vi "Configure Status.vi"(0 "disk streaming in":refnum<class "Disk Streaming.lvclass">, 1 "preview size (samples)":u32, 5 "error in (no error)":errorcluster) -> (14 "disk streaming out":refnum<class "Disk Streaming.lvclass">, 19 "error out":errorcluster)   [LabVIEW 2021, in "Disk Streaming.lvclass"]
doc: "Configures the status properties of a disk streaming instance. For more information about the disk streaming instance refer to the <B>Open.vi</B> context help.\n\nInputs:\n\n<B>disk streaming in</B>: Disk streaming instance input.\n\n<B>preview size (samples)</B>: The desired preview size, in samples. The preview is a snapshot of the recently streamed samples, a small part of the sample sequence transferred between the disk and the FPGA Target. The preview is updated only on <B>Read</B> and <B>Write</B> VI calls, and it can be obtained using the <B>Get Status.vi</B>.\n\nOutputs:\n\n<B>disk streaming out</B>: Disk streaming instance output. Pass this output to the other Disk Streaming VIs to perform the streaming."
uses:
  Disk Streaming.lvclass
  Disk Streaming.lvclass/Disk Streaming.ctl
  Private/Command.ctl
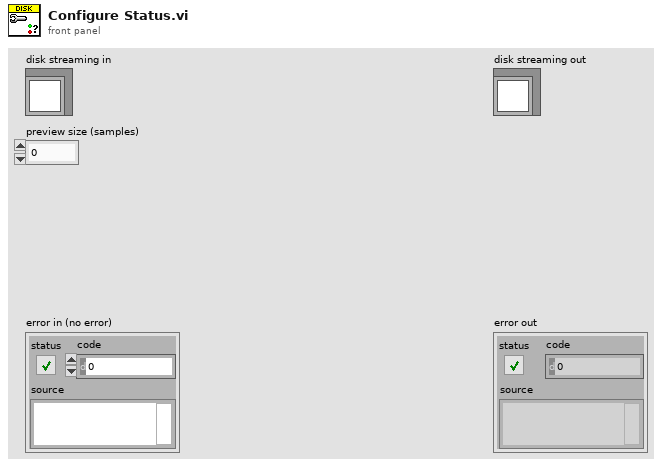
[diagram p1: front panel]
types:
  T1 = typedef "Disk Streaming.lvclass/Command.ctl" = cluster{"preview size":i32}
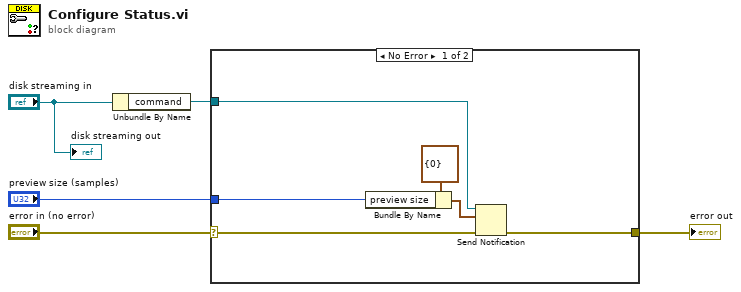
[diagram p0: block diagram]
diagram:
  n1 = Unbundle By Name("disk streaming in") -> ("command"=w1:refnum<notifier>)
  n2 = case shown="No Error" "error in (no error)" {
    selector: "error in (no error)" -> [w8 w12]
    tunnel: [w6 w12] -> w4
    tunnel: "preview size (samples)" -> [w7 _]
    tunnel: w1 -> [w11 _]
    frame No Error {
      n3 = Bundle By Name(cluster=T1 {"preview size"=0} ("Disk Streaming Descriptor Command"), "preview size"=w7) -> (w9:T1)
      n4 = Send Notification(notification=w9, notifier=w11, error in (no error)=w8) -> (error out=w6:errorcluster)  [unwired: 1 out]
    }
    frame Error {
    }
  }
  "error out" <- w4
  "disk streaming out" <- "disk streaming in"
